vi "XIPIN_1G_2.5G_Ethernet_PCS_PMA_or_SGMII_15_1.vi"   [LabVIEW 2017]
doc: "The 1G/2.5G Ethernet PCS/PMA or SGMII LogiCORE(TM) provides the functionality to implement one of two different specifications: firstly the IEEE 802.3 1000BASE-X specification; secondly the Serial-GMII (SGMII) specification which is closely based on 1000BASE-X. The core provides a choice of physical interface options: a Ten-Bit-Interface (TBI) for connection to an external SERDES; high speed serial functionality using the device specific transceivers in Virtex-7, Kintex-7 and Artix-7; SGMII standard only - LVDS using SelectIO in Kintex-7 devices -2 speed grade and faster. All options provide up to 1/2.5 gigabit per second total bandwidth. When perfoming the SGMII standard, the core can carry Ethernet traffic up to 1/2.5 gigabit per second total bandwidth; this is inclusive of 10Mbps, 100Mbps, 1Gbps and 2.5Gbps Ethernet speeds. The core is designed to interface to the LogiCORE Tri-Mode Ethernet MAC or Zynq Processor subsystem from Xilinx to provide a complete solution.\n------------------------------------\n<b>Need License</b> : No"
uses:
  <vilib>/rvi/XilinxIP/XIPIN_XNode/niFpgaXIPIN.xnode
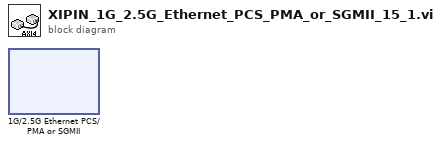
[diagram p0: block diagram]
diagram:
  n1 = xnode ("1G/2.5G Ethernet PCS/PMA or SGMII")() -> ()
